vi "_Test_MM_Unit_test.vi"() -> ()   [LabVIEW 2023]
uses:
  MM/MM.lvlib
panel:
  out "Array 3":i32[](array[numeric])
  out "error out":errorcluster
  out "simFrame":dbl
  out "simTime":dbl
  out "Array 2":u8[](array[numeric])
  out "Array":string[](array[string])
  in  "file path (use dialog)":path=path "C:/Debug/debug_MM_Package_error"
  in  "path in":path=path "C:/dev/Hexagon-VTD-Custom-Device/Libraries/libMM.dll"
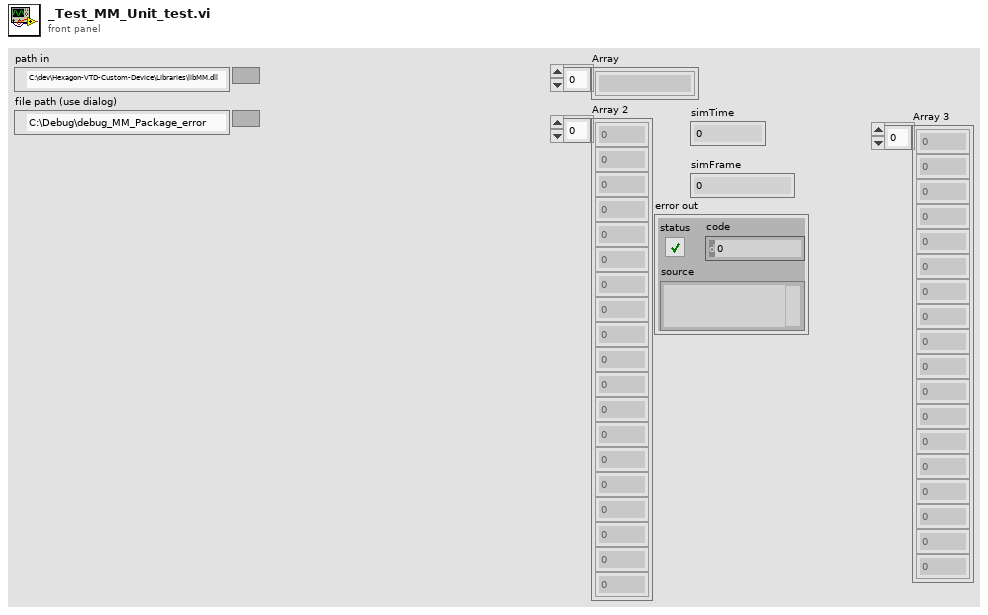
[diagram p1: front panel]
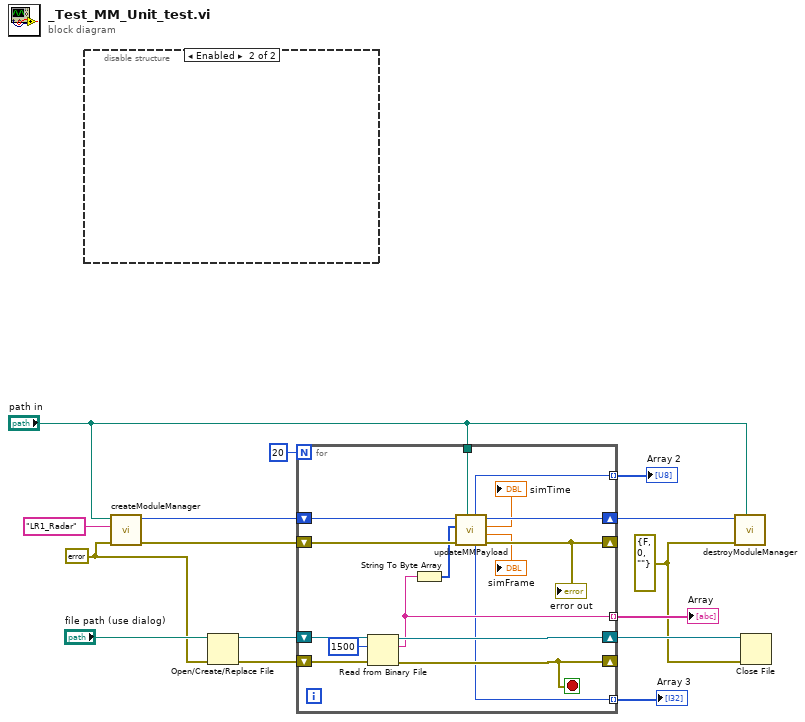
[diagram p0: block diagram]
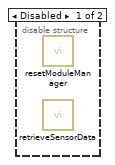
[diagram p2: hidden frame]
diagram:
  w2 = errorcluster {"status"=FALSE, "code"=0, "source"=""} ("error in (no error)")
  w6 = errorcluster {"status"=FALSE, "code"=0, "source"=""} ("error in (no error)")
  n1 = disable-structure shown="Enabled" {
    frame Disabled {
      n2 = call "resetModuleManager.vi"() -> ()  [unwired: 11 in, 1 out]
      n3 = call "retrieveSensorData.vi"() -> ()  [unwired: 13 in, 3 out]
    }
    frame Enabled {
    }
  }
  n4 = call "createModuleManager.vi"("error in (no error)"=w6, "sensorName"="LR1_Radar", "path in"="path in") -> ("error out"=w14:errorcluster, "mmHandle"=w15:u64)  [unwired: 7 in]
  n5 = Open/Create/Replace File(file path (use dialog)="file path (use dialog)", error in=w6) -> (refnum out=w10:refnum<file>, error out=w9:errorcluster)  [unwired: 4 in, 1 out]
  n6 = for {
    N: 20 -> [_]
    tunnel: "path in" -> [w27]
    shift-right: [w29] -> w13
    shift-left: w15 -> [w31]
    shift-right: [w28] -> _
    shift-left: w14 -> [w30]
    shift-right: [w24] -> w8
    shift-left: w10 -> [w26]
    shift-right: [w21] -> _
    shift-left: w9 -> [w25]
    tunnel: [w20] -> w5 mode=indexing
    tunnel: [w19] -> w4 mode=indexing
    tunnel: [w16] -> w1 mode=indexing
    stop <- w21 stop-if-true
    n7 = Read from Binary File(8:w25, 10:1500 ("count (1)"), 11:w26) -> (0:w21:errorcluster, 2:w20:string, 3:w24:refnum<file>)  [unwired: 3 in, 1 out]
    n8 = String To Byte Array(string=w20) -> (unsigned byte array=w22:u8[])
    n9 = call "updateMMPayload.vi"("path in"=w27, "error in (no error)"=w30, "payload"=w22, "mmHandle in"=w31) -> ("error out"=w28:errorcluster, "simFrame"=→"simFrame":dbl, "simTime"=→"simTime":dbl, "mmHandle out"=w29:u64, "return type"=w16:i32, "isComplete"=w19:u8)  [unwired: 2 in]
    "error out" <- w28
  }
  "Array" <- w5
  "Array 2" <- w4
  "Array 3" <- w1
  n10 = call "destroyModuleManager.vi"("path in"="path in", "error in (no error)"=w2, "mmHandle"=w13) -> ()  [unwired: 8 in, 1 out]
  n11 = Close File(refnum=w8, error in=w2) -> ()  [unwired: 2 out]
